vi "rsscope_core_global.vi"() -> ()   [LabVIEW 2014] (continued)
"Read Callback"="", "Write Callback"="", "Supported Models"="", "Instrument Options"="", "Flags"=0, "Help"="Selects the operation type to be performed on the selected operands for the spectrum arithmetic measurement.\n\nAvailable Repeated Capabilities:\nMeasurement: Meas1, Meas2, Meas3, Meas4, Meas5, Meas6, Meas7, Meas8, Meas9, Meas10\r\n\nRemote-control command(s):\nMEASurement<m>:SPECtrum:ARIThmetic:OPERator"}, {"Level"=4, "Class Only"=FALSE, "Identifier"="RSSCOPE_ATTR_SPECTRUM_ARITHMETIC_CONSTANT", "Descriptive Name"="Spectrum Arithmetic Constant", "Data Type"=1, "Command"="MEAS{Measurement}:SPEC:ARIT:CONS", "Access"=2, "Range Table"="RsScope_rngArithmeticConstant", "Read Callback"="", "Write Callback"="", "Supported Models"="", "Instrument Options"="", "Flags"=0, "Help"="Sets a constant numeric value as the second operand of the spectrum arithmetic measurement.\n\nAvailable Repeated Capabilities:\nMeasurement: Meas1, Meas2, Meas3, Meas4, Meas5, Meas6, Meas7, Meas8, Meas9, Meas10\r\n\nRemote-control command(s):\nMEASurement<m>:SPECtrum:ARIThmetic:CONStant"}, {"Level"=4, "Class Only"=FALSE, "Identifier"="RSSCOPE_ATTR_SPECTRUM_ARITHMETIC_CONSTANT_UNIT", "Descriptive Name"="Spectrum Arithmetic Constant Unit", "Data Type"=0, "Command"="MEAS{Measurement}:SPEC:ARIT:COUN", "Access"=2, "Range Table"="RsScope_rngArithmeticOperationType", "Read Callback"="", "Write Callback"="", "Supported Models"="", "Instrument Options"="", "Flags"=0, "Help"="Selects the operation type to be performed on the selected operands for the amplitude/time arithmetic measurement.\n\nAvailable Repeated Capabilities:\nMeasurement: Meas1, Meas2, Meas3, Meas4, Meas5, Meas6, Meas7, Meas8, Meas9, Meas10\r\n\nRemote-control command(s):\nMEASurement<m>:SPECtrum:ARIThmetic:COUNit"}, {"Level"=4, "Class Only"=FALSE, "Identifier"="RSSCOPE_ATTR_SPECTRUM_ARITHMETIC_CUSTOM_NAME_ENABLED", "Descriptive Name"="Spectrum Arithmetic Custom Name Enabled", "Data Type"=3, "Command"="MEAS{Measurement}:SPEC:ARIT:CUNS", "Access"=2, "Range Table"="", "Read Callback"="", "Write Callback"="", "Supported Models"="", "Instrument Options"="", "Flags"=0, "Help"="Enables the use of user-defined custom name for the spectrum arithmetic measurement.\n\nAvailable Repeated Capabilities:\nMeasurement: Meas1, Meas2, Meas3, Meas4, Meas5, Meas6, Meas7, Meas8, Meas9, Meas10\r\n\nRemote-control command(s):\nMEASurement<m>:SPECtrum:ARIThmetic:CUNState"}, {"Level"=4, "Class Only"=FALSE, "Identifier"="RSSCOPE_ATTR_SPECTRUM_ARITHMETIC_CUSTOM_UNIT_ENABLED", "Descriptive Name"="Spectrum Arithmetic Custom Unit Enabled", "Data Type"=3, "Command"="MEAS{Measurement}:SPEC:ARIT:CUUS", "Access"=2, "Range Table"="", "Read Callback"="", "Write Callback"="", "Supported Models"="", "Instrument Options"="", "Flags"=0, "Help"="Enables the use of user-defined custom unit for the amplitude/time arithmetic measurement. You can set the unit with RSSCOPE_ATTR_SPECTRUM_ARITHMETIC_CUSTOM_UNIT.\n\nAvailable Repeated Capabilities:\nMeasurement: Meas1, Meas2, Meas3, Meas4, Meas5, Meas6, Meas7, Meas8, Meas9, Meas10\r\n\nRemote-control command(s):\nMEASurement<m>:SPECtrum:ARIThmetic:CUUState"}, {"Level"=4, "Class Only"=FALSE, "Identifier"="RSSCOPE_ATTR_SPECTRUM_ARITHMETIC_CUSTOM_UNIT", "Descriptive Name"="Spectrum Arithmetic Custom Unit", "Data Type"=2, "Command"="MEAS{Measurement}:SPEC:ARIT:CUUN", "Access"=2, "Range Table"="", "Read Callback"="", "Write Callback"="", "Supported Models"="", "Instrument Options"="", "Flags"=0, "Help"="Sets a user-defined value of the unit for the spectrum arithmetic measurement.\n\nAvailable Repeated Capabilities:\nMeasurement: Meas1, Meas2, Meas3, Meas4, Meas5, Meas6, Meas7, Meas8, Meas9, Meas10\r\n\nRemote-control command(s):\nMEASurement<m>:SPECtrum:ARIThmetic:CUUNit"}, {"Level"=2, "Class Only"=TRUE, "Identifier"="", "Descriptive Name"="Statistics And Long-term Measurement", "Data Type"=0, "Command"="", "Access"=0, "Range Table"="", "Read Callback"="", "Write Callback"="", "Supported Models"="", "Instrument Options"="", "Flags"=0, "Help"="Statistics And Long-term Measurement configures long term measurements, including statistics and measurement histogram over a longer period of time."}, {"Level"=3, "Class Only"=FALSE, "Identifier"="RSSCOPE_ATTR_STATISTICS_ENABLED", "Descriptive Name"="Statistics Enabled", "Data Type"=3, "Command"="MEAS{Measurement}:STAT", "Access"=2, "Range Table"="", "Read Callback"="", "Write Callback"="", "Supported Models"="", "Instrument Options"="", "Flags"=0, "Help"="Enables statistics calculation for the measurement. For RTE the statistics can only be switched globally for all measurements.\n\nAvailable Repeated Capabilities:\nMeasurement: Meas1, Meas2, Meas3, Meas4, Meas5, Meas6, Meas7, Meas8, Meas9, Meas10\r\n\nRemote-control command(s):\nMEASurement<m>:STATistics[:ENABle]"}, {"Level"=3, "Class Only"=FALSE, "Identifier"="RSSCOPE_ATTR_STATISTICS_HISTOGRAM_ENABLED", "Descriptive Name"="Statistics Histogram Enabled", "Data Type"=3, "Command"="MEAS{Measurement}:STAT:HIST", "Access"=2, "Range Table"="", "Read Callback"="", "Write Callback"="", "Supported Models"="", "Instrument Options"="", "Flags"=0, "Help"="Displays histogram of the statistical results. Enabling the histogram enables also the calculation and display of statistics for the measurement results if statistics were disabled. The histogram shows the cumulative occurence distribution of mean measurement results in a graphic.\n\nAvailable Repeated Capabilities:\nMeasurement: Meas1, Meas2, Meas3, Meas4, Meas5, Meas6, Meas7, Meas8, Meas9, Meas10\r\n\nRemote-control command(s):\nMEASurement<m>:STATistics:HISTogram"}, {"Level"=3, "Class Only"=FALSE, "Identifier"="RSSCOPE_ATTR_STATISTICS_RESET_MODE", "Descriptive Name"="Statistics Reset Mode", "Data Type"=0, "Command"="MEAS{Measurement}:STAT:MODE", "Access"=2, "Range Table"="rsscope_rngStatisticsMode", "Read Callback"="", "Write Callback"="", "Supported Models"="", "Instrument Options"="", "Flags"=0, "Help"="Defines when the statistics for long term measurements are reset.\n\nAvailable Repeated Capabilities:\nMeasurement: Meas1, Meas2, Meas3, Meas4, Meas5, Meas6, Meas7, Meas8, Meas9, Meas10\r\n\nRemote-control command(s):\nMEASurement<m>:STATistics:MODE"}, {"Level"=3, "Class Only"=FALSE, "Identifier"="RSSCOPE_ATTR_STATISTICS_RESET_COUNT", "Descriptive Name"="Statistics Reset Count", "Data Type"=0, "Command"="MEAS{Measurement}:STAT:RCO", "Access"=2, "Range Table"="rsscope_rngResetCount", "Read Callback"="", "Write Callback"="", "Supported Models"="", "Instrument Options"="", "Flags"=0, "Help"="Defines the number of measurements after which the statistics are reset.\n\nAvailable Repeated Capabilities:\nMeasurement: Meas1, Meas2, Meas3, Meas4, Meas5, Meas6, Meas7, Meas8, Meas9, Meas10\r\n\nRemote-control command(s):\nMEASurement<m>:STATistics:RCOunt"}, {"Level"=3, "Class Only"=FALSE, "Identifier"="RSSCOPE_ATTR_STATISTICS_RESET_TIME", "Descriptive Name"="Statistics Reset Time", "Data Type"=1, "Command"="MEAS{Measurement}:STAT:RTIM", "Access"=2, "Range Table"="rsscope_rngResetTime", "Read Callback"="", "Write Callback"="", "Supported Models"="", "Instrument Options"="", "Flags"=0, "Help"="Defines the time or period after which the statistics are reset.\n\nAvailable Repeated Capabilities:\nMeasurement: Meas1, Meas2, Meas3, Meas4, Meas5, Meas6, Meas7, Meas8, Meas9, Meas10\r\n\nRemote-control command(s):\nMEASurement<m>:STATistics:RTIMe"}, {"Level"=3, "Class Only"=FALSE, "Identifier"="RSSCOPE_ATTR_STATISTICS_RESET_MEASUREMENTS_COUNT", "Descriptive Name"="Statistics Reset Measurements Count", "Data Type"=0, "Command"="MEAS{Measurement}:STAT:RME", "Access"=2, "Range Table"="rsscope_rngStatisticsMeasurementsCount", "Read Callback"="", "Write Callback"="", "Supported Models"="", "Instrument Options"="", "Flags"=0, "Help"="Defines the number of measurement results from which one point of the long term measurement is created.\n\nAvailable Repeated Capabilities:\nMeasurement: Meas1, Meas2, Meas3, Meas4, Meas5, Meas6, Meas7, Meas8, Meas9, Meas10\r\n\nRemote-control command(s):\nMEASurement<m>:STATistics:RMEascount"}, {"Level"=3, "Class Only"=FALSE, "Identifier"="RSSCOPE_ATTR_STATISTICS_RESET", "Descriptive Name"="Statistics Reset", "Data Type"=4, "Command"="MEAS{Measurement}:STAT:RES", "Access"=1, "Range Table"="", "Read Callback"="", "Write Callback"="", "Supported Models"="", "Instrument Options"="", "Flags"=0, "Help"="Resets the statistics.\n\nAvailable Repeated Capabilities:\nMeasurement: Meas1, Meas2, Meas3, Meas4, Meas5, Meas6, Meas7, Meas8, Meas9, Meas10\r\n\nRemote-control command(s):\nMEASurement<m>:STATistics:RESet"}, {"Level"=3, "Class Only"=FALSE, "Identifier"="RSSCOPE_ATTR_STATISTICS_NUMBER_OF_BINS", "Descriptive Name"="Statistics Number Of Bins", "Data Type"=0, "Command"="MEAS{Measurement}:STAT:HBIN", "Access"=2, "Range Table"="RsScope_rngStatisticsNumberOfBins", "Read Callback"="", "Write Callback"="", "Supported Models"="", "Instrument Options"="", "Flags"=0, "Help"="Sets the number of bins - the number of vertical bars that build the histogram. If &apos;Continuous auto scale&apos; is enabled, the instrument determines the number of bins based on the time base, the current measurements, and other settings. To set the number of bins manually, disable &apos;Continuous auto scale&apos;.\n\nAvailable Repeated Capabilities:\nMeasurement: Meas1, Meas2, Meas3, Meas4, Meas5, Meas6, Meas7, Meas8, Meas9, Meas10\r\n\nRemote-control command(s):\nMEASurement<m>:STATistics:HBINs"}, {"Level"=3, "Class Only"=FALSE, "Identifier"="RSSCOPE_ATTR_TRACK_ENABLED", "Descriptive Name"="Track Enabled", "Data Type"=3, "Command"="MEAS{Measurement}:TRAC", "Access"=2, "Range Table"="", "Read Callback"="", "Write Callback"="", "Supported Models"="", "Instrument Options"="", "Flags"=0, "Help"="Enables or disables the track of the indicated channel.\n\nAvailable Repeated Capabilities:\nMeasurement: Meas1, Meas2, Meas3, Meas4, Meas5, Meas6, Meas7, Meas8, Meas9, Meas10\r\n\nRemote-control command(s):\nMEASurement<m>:TRACk[:STATe]"}, {"Level"=3, "Class Only"=FALSE, "Identifier"="RSSCOPE_ATTR_PROTOCOL_AUDIO_TRACK_ENABLED", "Descriptive Name"="Protocol Audio Track Enabled", "Data Type"=3, "Command"="MEAS{Measurement}:TRAC", "Access"=2, "Range Table"="", "Read Callback"="", "Write Callback"="", "Supported Models"="", "Instrument Options"="", "Flags"=0, "Help"="Enables or disables the track of the indicated channel.\n\nAvailable Repeated Capabilities:\nMeasurement: Meas1, Meas2, Meas3, Meas4, Meas5, Meas6, Meas7, Meas8, Meas9, Meas10\r\n\nRemote-control command(s):\nMEASurement<m>:TRACk[:STATe]"}, {"Level"=3, "Class Only"=FALSE, "Identifier"="RSSCOPE_ATTR_TRACK_WAVEFORM_HEADER", "Descriptive Name"="Track Waveform Header", "Data Type"=2, "Command"="MEAS{Measurement}:TRAC:DATA:HEAD?", "Access"=0, "Range Table"="", "Read Callback"="", "Write Callback"="", "Supported Models"="", "Instrument Options"="", "Flags"=0, "Help"="Returns the header of the track.\n\nAvailable Repeated Capabilities:\nMeasurement: Meas1, Meas2, Meas3, Meas4, Meas5, Meas6, Meas7, Meas8, Meas9, Meas10\r\n\nRemote-control command(s):\nMEASurement<m>:TRACk:DATA:HEADer?"}, {"Level"=3, "Class Only"=FALSE, "Identifier"="RSSCOPE_ATTR_TRACK_WAVEFORM_DATA_TYPE", "Descriptive Name"="Track Waveform Data Type", "Data Type"=2, "Command"="MEAS{Measurement}:TRAC:DATA:STYP?", "Access"=0, "Range Table"="", "Read Callback"="", "Write Callback"="", "Supported Models"="", "Instrument Options"="", "Flags"=0, "Help"="Returns the data type.\n\nAvailable Repeated Capabilities:\nMeasurement: Meas1, Meas2, Meas3, Meas4, Meas5, Meas6, Meas7, Meas8, Meas9, Meas10\r\n\nRemote-control command(s):\nMEASurement<m>:TRACk:DATA:STYPe?"}, {"Level"=3, "Class Only"=FALSE, "Identifier"="RSSCOPE_ATTR_PROTOCOL_AUDIO_TRACK_WAVEFORM_DATA_TYPE", "Descriptive Name"="Protocol Audio Track Waveform Data Type", "Data Type"=2, "Command"="MEAS{Measurement}:TRAC:DATA:STYP?", "Access"=0, "Range Table"="", "Read Callback"="", "Write Callback"="", "Supported Models"="", "Instrument Options"="", "Flags"=0, "Help"="Returns the data type.\n\nAvailable Repeated Capabilities:\nMeasurement: Meas1, Meas2, Meas3, Meas4, Meas5, Meas6, Meas7, Meas8, Meas9, Meas10\r\n\nRemote-control command(s):\nMEASurement<m>:TRACk:DATA:STYPe?"}, {"Level"=3, "Class Only"=FALSE, "Identifier"="RSSCOPE_ATTR_LONG_TERM_MEASUREMENT_ENABLED", "Descriptive Name"="Long Term Measurement Enabled", "Data Type"=3, "Command"="MEAS{Measurement}:LTM", "Access"=2, "Range Table"="", "Read Callback"="", "Write Callback"="", "Supported Models"="", "Instrument Options"="", "Flags"=0, "Help"="Enables long term measurement for a defined number of measurement points or a specified time.\n\nAvailable Repeated Capabilities:\nMeasurement: Meas1, Meas2, Meas3, Meas4, Meas5, Meas6, Meas7, Meas8, Meas9, Meas10\r\n\nRemote-control command(s):\nMEASurement<m>:LTMeas[:STATe]"}, {"Level"=3, "Class Only"=FALSE, "Identifier"="RSSCOPE_ATTR_LONG_TERM_COUNT", "Descriptive Name"="Long Term Count", "Data Type"=0, "Command"="MEAS{Measurement}:LTM:COUN", "Access"=2, "Range Table"="rsscope_rngLongTermCount", "Read Callback"="", "Write Callback"="", "Supported Models"="", "Instrument Options"="", "Flags"=0, "Help"="Defines the total number of points to be measured during the long term measurement.\n\nAvailable Repeated Capabilities:\nMeasurement: Meas1, Meas2, Meas3, Meas4, Meas5, Meas6, Meas7, Meas8, Meas9, Meas10\r\n\nRemote-control command(s):\nMEASurement<m>:LTMeas:COUNt"}, {"Level"=3, "Class Only"=FALSE, "Identifier"="RSSCOPE_ATTR_LONG_TERM_DURATION", "Descriptive Name"="Long Term Duration", "Data Type"=0, "Command"="MEAS{Measurement}:LTM:TIME", "Access"=2, "Range Table"="", "Read Callback"="", "Write Callback"="", "Supported Models"="", "Instrument Options"="", "Flags"=0, "Help"="Defines the total duration of the long term measurement.\n\nAvailable Repeated Capabilities:\nMeasurement: Meas1, Meas2, Meas3, Meas4, Meas5, Meas6, Meas7, Meas8, Meas9, Meas10\r\n\nRemote-control command(s):\nMEASurement<m>:LTMeas:TIME"}, {"Level"=3, "Class Only"=FALSE, "Identifier"="RSSCOPE_ATTR_LONG_TERM_VERTICAL_OFFSET", "Descriptive Name"="Long Term Vertical Offset", "Data Type"=1, "Command"="MEAS{Measurement}:VERT:OFFS", "Access"=2, "Range Table"="", "Read Callback"="", "Write Callback"="", "Supported Models"="", "Instrument Options"="", "Flags"=0, "Help"="Defines a vertical offset for the long term measurement.\n\nAvailable Repeated Capabilities:\nMeasurement: Meas1, Meas2, Meas3, Meas4, Meas5, Meas6, Meas7, Meas8, Meas9, Meas10\r\n\nRemote-control command(s):\nMEASurement<m>:VERTical:OFFSet"}, {"Level"=3, "Class Only"=FALSE, "Identifier"="RSSCOPE_ATTR_LONG_TERM_VERTICAL_SCALING", "Descriptive Name"="Long Term Vertical Scaling", "Data Type"=1, "Command"="MEAS{Measurement}:VERT:SCAL", "Access"=2, "Range Table"="RsScope_rngLongTermVerticalScaling", "Read Callback"="", "Write Callback"="", "Supported Models"="", "Instrument Options"="", "Flags"=0, "Help"="Defines the vertical scaling per division, so that the scaling can be adapted automatically during the long term measurement period.\n\nAvailable Repeated Capabilities:\nMeasurement: Meas1, Meas2, Meas3, Meas4, Meas5, Meas6, Meas7, Meas8, Meas9, Meas10\r\n\nRemote-control command(s):\nMEASurement<m>:VERTical:SCALe"}, {"Level"=3, "Class Only"=FALSE, "Identifier"="RSSCOPE_ATTR_LONG_TERM_VERTICAL_CONTINUOUS_AUTO_SCALING", "Descriptive Name"="Long Term Vertical Continuous Auto Scaling", "Data Type"=3, "Command"="MEAS{Measurement}:VERT:CONT", "Access"=2, "Range Table"="", "Read Callback"="", "Write Callback"="", "Supported Models"="", "Instrument Options"="", "Flags"=0, "Help"="If enabled, automatic vertical scaling is performed whenever the waveform does not fit in the diagram during the long term measurement period.\n\nAvailable Repeated Capabilities:\nMeasurement: Meas1, Meas2, Meas3, Meas4, Meas5, Meas6, Meas7, Meas8, Meas9, Meas10\r\n\nRemote-control command(s):\nMEASurement<m>:VERTical:CONT"}, {"Level"=3, "Class Only"=FALSE, "Identifier"="RSSCOPE_ATTR_LONG_TERM_VERTICAL_AUTOSCALE", "Descriptive Name"="Long Term Vertical Autoscale", "Data Type"=4, "Command"="MEAS{Measurement}:VERT:AUTO", "Access"=1, "Range Table"="", "Read Callback"="", "Write Callback"="", "Supported Models"="", "Instrument Options"="", "Flags"=0, "Help"="If enabled, vertical scaling is adapted to the current measurement results automatically during the long term measurement period.\n\nAvailable Repeated Capabilities:\nMeasurement: Meas1, Meas2, Meas3, Meas4, Meas5, Meas6, Meas7, Meas8, Meas9, Meas10\r\n\nRemote-control command(s):\nMEASurement<m>:VERTical:AUTO"}, {"Level"=3, "Class Only"=FALSE, "Identifier"="RSSCOPE_ATTR_LONG_TERM_ENVIRONMENT_SENSOR_ENABLED", "Descriptive Name"="Long Term Environment Sensor Enabled", "Data Type"=3, "Command"="MEAS{Measurement}:LTM:ENVS:STAT", "Access"=2, "Range Table"="", "Read Callback"="", "Write Callback"="", "Supported Models"="", "Instrument Options"="", "Flags"=0, "Help"="Enables the evaluation of a connected environment sensor.\n\nAvailable Repeated Capabilities:\nMeasurement: Meas1, Meas2, Meas3, Meas4, Meas5, Meas6, Meas7, Meas8, Meas9, Meas10\r\n\nRemote-control command(s):\nMEASurement<m>:LTMeas:ENVSensor:STATe"}, {"Level"=2, "Class Only"=TRUE, "Identifier"="", "Descriptive Name"="Protocol", "Data Type"=0, "Command"="", "Access"=0, "Range Table"="", "Read Callback"="", "Write Callback"="", "Supported Models"="", "Instrument Options"="", "Flags"=0, "Help"="This class contains methods for configuring and measuring protocol measurements. Before starting the protocol measurement a bus type has to be selected (RSSCOPE_ATTR_PROTOCOL_TYPE) and the bus has to be activated (RSSCOPE_ATTR_PROTOCOL_STATE)."}, {"Level"=3, "Class Only"=FALSE, "Identifier"="RSSCOPE_ATTR_PROTOCOL_MAIN_MEASUREMENT", "Descriptive Name"="Protocol Main Measurement", "Data Type"=0, "Command"="MEAS{Measurement}:MAIN", "Access"=2, "Range Table"="rsscope_rngProtocolMeasurementType", "Read Callback"="", "Write Callback"="", "Supported Models"="", "Instrument Options"="K35", "Flags"=0, "Help"="Defines or queries the main measurement. This measurement is the one referred to if the measurement waveform is used as a source for math calculations. The main measurement type must belong to the same category as the other types assigned to the same measurement waveform, if there are any.\n\nAvailable Repeated Capabilities:\nMeasurement: Meas1, Meas2, Meas3, Meas4, Meas5, Meas6, Meas7, Meas8, Meas9, Meas10\r\n\nRemote-control command(s):\nMEASurement<m>:MAIN"}, {"Level"=3, "Class Only"=FALSE, "Identifier"="RSSCOPE_ATTR_PROTOCOL_ADDITIONAL_MEASUREMENT", "Descriptive Name"="Protocol Additional Measurement", "Data Type"=6, "Command"="MEAS{Measurement}:ADD", "Access"=1, "Range Table"="", "Read Callback"="", "Write Callback"="", "Supported Models"="", "Instrument Options"="K35", "Flags"=0, "Help"="Adds additional measurements to the indicated measurement group. Only one measurement can be enabled or disabled per command. The query returns the state of the specified measurement.\n\nNote that each measurement group must contain measurements from the same category. For example, if the main measurement of measurement group 1 is amplitude, then you cannot enable an eye width measurementin the same measurement group.\n\nAvailable Repeated Capabilities:\nMeasurement: Meas1, Meas2, Meas3, Meas4, Meas5, Meas6, Meas7, Meas8, Meas9, Meas10\r\n\nRemote-control command(s):\nMEASurement<m>:ADDitional"}, {"Level"=3, "Class Only"=FALSE, "Identifier"="RSSCOPE_ATTR_FRAME_TO_FRAME_FROM_FRAME", "Descriptive Name"="Frame To Frame From Frame", "Data Type"=2, "Command"="MEAS{Measurement}:PROT:F2FR:FRMF", "Access"=2, "Range Table"="", "Read Callback"="", "Write Callback"="", "Supported Models"="", "Instrument Options"="", "Flags"=0, "Help"="Sets the type of start frame for the frame to frame protocol measurement. Valid values vary by protocol.\n\nAvailable Repeated Capabilities:\nMeasurement: Meas1, Meas2, Meas3, Meas4, Meas5, Meas6, Meas7, Meas8, Meas9, Meas10\r\n\nRemote-control command(s):\nMEASurement<m>:PROTocol:F2FRame:FRMFrom"}, {"Level"=3, "Class Only"=FALSE, "Identifier"="RSSCOPE_ATTR_FRAME_TO_FRAME_FROM_FIELD", "Descriptive Name"="Frame To Frame From Field", "Data Type"=2, "Command"="MEAS{Measurement}:PROT:F2FR:FLDF", "Access"=2, "Range Table"="", "Read Callback"="", "Write Callback"="", "Supported Models"="", "Instrument Options"="", "Flags"=0, "Help"="Sets the type of field for the start frame of the frame to frame protocol measurement. Valid values vary by frame.\n\nAvailable Repeated Capabilities:\nMeasurement: Meas1, Meas2, Meas3, Meas4, Meas5, Meas6, Meas7, Meas8, Meas9, Meas10\r\n\nRemote-control command(s):\nMEASurement<m>:PROTocol:F2FRame:FLDFrom"}, {"Level"=3, "Class Only"=FALSE, "Identifier"="RSSCOPE_ATTR_FRAME_TO_FRAME_FROM_VALUE", "Descriptive Name"="Frame To Frame From Value", "Data Type"=2, "Command"="MEAS{Measurement}:PROT:F2FR:VALF", "Access"=2, "Range Table"="", "Read Callback"="", "Write Callback"="", "Supported Models"="", "Instrument Options"="", "Flags"=0, "Help"="Sets the field value of the start frame for the frame to frame protocol measurement.\n\nAvailable Repeated Capabilities:\nMeasurement: Meas1, Meas2, Meas3, Meas4, Meas5, Meas6, Meas7, Meas8, Meas9, Meas10\r\n\nRemote-control command(s):\nMEASurement<m>:PROTocol:F2FRame:VALFrom"}, {"Level"=3, "Class Only"=FALSE, "Identifier"="RSSCOPE_ATTR_FRAME_TO_FRAME_TO_FRAME", "Descriptive Name"="Frame To Frame To Frame", "Data Type"=2, "Command"="MEAS{Measurement}:PROT:F2FR:FRMT", "Access"=2, "Range Table"="", "Read Callback"="", "Write Callback"="", "Supported Models"="", "Instrument Options"="", "Flags"=0, "Help"="Sets the type of end frame for the frame to frame protocol measurement. Valid values vary by protocol.\n\nAvailable Repeated Capabilities:\nMeasurement: Meas1, Meas2, Meas3, Meas4, Meas5, Meas6, Meas7, Meas8, Meas9, Meas10\r\n\nRemote-control command(s):\nMEASurement<m>:PROTocol:F2FRame:FRMTo"}, {"Level"=3, "Class Only"=FALSE, "Identifier"="RSSCOPE_ATTR_FRAME_TO_FRAME_TO_FIELD", "Descriptive Name"="Frame To Frame To Field", "Data Type"=2, "Command"="MEAS{Measurement}:PROT:F2FR:FLDT", "Access"=2, "Range Table"="", "Read Callback"="", "Write Callback"="", "Supported Models"="", "Instrument Options"="", "Flags"=0, "Help"="Sets the type of field for the end frame of the frame to frame protocol measurement. Valid values vary by frame.\n\nAvailable Repeated Capabilities:\nMeasurement: Meas1, Meas2, Meas3, Meas4, Meas5, Meas6, Meas7, Meas8, Meas9, Meas10\r\n\nRemote-control command(s):\nMEASurement<m>:PROTocol:F2FRame:FLDTo"}, {"Level"=3, "Class Only"=FALSE, "Identifier"="RSSCOPE_ATTR_FRAME_TO_FRAME_TO_VALUE", "Descriptive Name"="Frame To Frame To Value", "Data Type"=2, "Command"="MEAS{Measurement}:PROT:F2FR:VALT", "Access"=2, "Range Table"="", "Read Callback"="", "Write Callback"="", "Supported Models"="", "Instrument Options"="", "Flags"=0, "Help"="Sets the field value of the end frame for the frame to frame protocol measurement.\n\nAvailable Repeated Capabilities:\nMeasurement: Meas1, Meas2, Meas3, Meas4, Meas5, Meas6, Meas7, Meas8, Meas9, Meas10\r\n\nRemote-control command(s):\nMEASurement<m>:PROTocol:F2FRame:VALTo"}, {"Level"=3, "Class Only"=FALSE, "Identifier"="RSSCOPE_ATTR_TRIGGER_TO_FRAME_DIRECTION", "Descriptive Name"="Trigger To Frame Direction", "Data Type"=0, "Command"="MEAS{Measurement}:PROT:T2FR:DIR", "Access"=2, "Range Table"="RsScope_rngTriggerToFrameDirection", "Read Callback"="", "Write Callback"="", "Supported Models"="", "Instrument Options"="", "Flags"=0, "Help"="Sets the direction of the field for trigger to frame protocol measurement.\n\nAvailable Repeated Capabilities:\nMeasurement: Meas1, Meas2, Meas3, Meas4, Meas5, Meas6, Meas7, Meas8, Meas9, Meas10\r\n\nRemote-control command(s):\nMEASurement<m>:PROTocol:T2FRame:DIRection"}, {"Level"=3, "Class Only"=FALSE, "Identifier"="RSSCOPE_ATTR_TRIGGER_TO_FRAME_FRAME", "Descriptive Name"="Trigger To Frame Frame", "Data Type"=2, "Command"="MEAS{Measurement}:PROT:T2FR:FRM", "Access"=2, "Range Table"="", "Read Callback"="", "Write Callback"="", "Supported Models"="", "Instrument Options"="", "Flags"=0, "Help"="Sets the value of the frame for trigger to frame protocol measurement. Valid values vary by protocol.\n\nAvailable Repeated Capabilities:\nMeasurement: Meas1, Meas2, Meas3, Meas4, Meas5, Meas6, Meas7, Meas8, Meas9, Meas10\r\n\nRemote-control command(s):\nMEASurement<m>:PROTocol:T2FRame:FRM"}, {"Level"=3, "Class Only"=FALSE, "Identifier"="RSSCOPE_ATTR_TRIGGER_TO_FRAME_FIELD", "Descriptive Name"="Trigger To Frame Field", "Data Type"=2, "Command"="MEAS{Measurement}:PROT:T2FR:FLD", "Access"=2, "Range Table"="", "Read Callback"="", "Write Callback"="", "Supported Models"="", "Instrument Options"="", "Flags"=0, "Help"="Sets the type of the field for trigger to frame protocol measurement. Valid values vary by frame.\n\nAvailable Repeated Capabilities:\nMeasurement: Meas1, Meas2, Meas3, Meas4, Meas5, Meas6, Meas7, Meas8, Meas9, Meas10\r\n\nRemote-control command(s):\nMEASurement<m>:PROTocol:T2FRame:FLD"}, {"Level"=3, "Class Only"=FALSE, "Identifier"="RSSCOPE_ATTR_TRIGGER_TO_FRAME_VALUE", "Descriptive Name"="Trigger To Frame Value", "Data Type"=2, "Command"="MEAS{Measurement}:PROT:T2FR:VAL", "Access"=2, "Range Table"="", "Read Callback"="", "Write Callback"="", "Supported Models"="", "Instrument Options"="", "Flags"=0, "Help"="Sets the value of the field for trigger to frame protocol measurement.\n\nAvailable Repeated Capabilities:\nMeasurement: Meas1, Meas2, Meas3, Meas4, Meas5, Meas6, Meas7, Meas8, Meas9, Meas10\r\n\nRemote-control command(s):\nMEASurement<m>:PROTocol:T2FRame:VALue"}, {"Level"=3, "Class Only"=FALSE, "Identifier"="RSSCOPE_ATTR_FIELD_VALUE_FRAME_IDENTIFICATION_FRAME", "Descriptive Name"="Field Value Frame Identification Frame", "Data Type"=2, "Command"="MEAS{Measurement}:PROT:FLDV:FRM", "Access"=2, "Range Table"="", "Read Callback"="", "Write Callback"="", "Supported Models"="", "Instrument Options"="", "Flags"=0, "Help"="Sets the type frame for the field value protocol measurement. Valid values vary by protocol.\n\nAvailable Repeated Capabilities:\nMeasurement: Meas1, Meas2, Meas3, Meas4, Meas5, Meas6, Meas7, Meas8, Meas9, Meas10\r\n\nRemote-control command(s):\nMEASurement<m>:PROTocol:FLDValue:FRM"}, {"Level"=3, "Class Only"=FALSE, "Identifier"="RSSCOPE_ATTR_FIELD_VALUE_FRAME_IDENTIFICATION_FIELD", "Descriptive Name"="Field Value Frame Identification Field", "Data Type"=2, "Command"="MEAS{Measurement}:PROT:FLDV:FLD", "Access"=2, "Range Table"="", "Read Callback"="", "Write Callback"="", "Supported Models"="", "Instrument Options"="", "Flags"=0, "Help"="Sets the type of field for the frame of the field value protocol measurement. Valid values vary by frame.\n\nAvailable Repeated Capabilities:\nMeasurement: Meas1, Meas2, Meas3, Meas4, Meas5, Meas6, Meas7, Meas8, Meas9, Meas10\r\n\nRemote-control command(s):\nMEASurement<m>:PROTocol:FLDValue:FLD"}, {"Level"=3, "Class Only"=FALSE, "Identifier"="RSSCOPE_ATTR_FIELD_VALUE_FRAME_IDENTIFICATION_VALUE", "Descriptive Name"="Field Value Frame Identification Value", "Data Type"=2, "Command"="MEAS{Measurement}:PROT:FLDV:VAL", "Access"=2, "Range Table"="", "Read Callback"="", "Write Callback"="", "Supported Models"="", "Instrument Options"="", "Flags"=0, "Help"="Sets the field value of the frame for the field value protocol measurement.\n\nAvailable Repeated Capabilities:\nMeasurement: Meas1, Meas2, Meas3, Meas4, Meas5, Meas6, Meas7, Meas8, Meas9, Meas10\r\n\nRemote-control command(s):\nMEASurement<m>:PROTocol:FLDValue:VALue"}, {"Level"=3, "Class Only"=FALSE, "Identifier"="RSSCOPE_ATTR_FIELD_VALUE_FIELD_TO_BE_TRACKED", "Descriptive Name"="Field Value Field To Be Tracked", "Data Type"=2, "Command"="MEAS{Measurement}:PROT:FLDV:TRCK", "Access"=2, "Range Table"="", "Read Callback"="", "Write Callback"="", "Supported Models"="", "Instrument Options"="", "Flags"=0, "Help"="Sets the field to be tracked value of the frame for the field value protocol measurement.\n\nAvailable Repeated Capabilities:\nMeasurement: Meas1, Meas2, Meas3, Meas4, Meas5, Meas6, Meas7, Meas8, Meas9, Meas10\r\n\nRemote-control command(s):\nMEASurement<m>:PROTocol:FLDValue:TRCK"}, {"Level"=3, "Class Only"=FALSE, "Identifier"="RSSCOPE_ATTR_MAIN_BIT_RATE_FRAME_NAME", "Descriptive Name"="Main Bit Rate Frame Name", "Data Type"=2, "Command"="MEAS{Measurement}:PROT:MBIT:FRM", "Access"=2, "Range Table"="", "Read Callback"="", "Write Callback"="", "Supported Models"="", "Instrument Options"="", "Flags"=0, "Help"="Sets the type frame for the main bit rate protocol measurement.\n\nAvailable Repeated Capabilities:\nMeasurement: Meas1, Meas2, Meas3, Meas4, Meas5, Meas6, Meas7, Meas8, Meas9, Meas10\r\n\nRemote-control command(s):\nMEASurement<m>:PROTocol:MBITrate:FRM"}, {"Level"=3, "Class Only"=FALSE, "Identifier"="RSSCOPE_ATTR_MAIN_BIT_RATE_FIELD_NAME", "Descriptive Name"="Main Bit Rate Field Name", "Data Type"=2, "Command"="MEAS{Measurement}:PROT:MBIT:FLD", "Access"=2, "Range Table"="", "Read Callback"="", "Write Callback"="", "Supported Models"="", "Instrument Options"="", "Flags"=0, "Help"="Sets the type of field for the frame of the main bit rate protocol measurement.\n\nAvailable Repeated Capabilities:\nMeasurement: Meas1, Meas2, Meas3, Meas4, Meas5, Meas6, Meas7, Meas8, Meas9, Meas10\r\n\nRemote-control command(s):\nMEASurement<m>:PROTocol:MBITrate:FLD"}, {"Level"=3, "Class Only"=FALSE, "Identifier"="RSSCOPE_ATTR_MAIN_BIT_RATE_ID_VALUE", "Descriptive Name"="Main Bit Rate ID Value", "Data Type"=6, "Command"="MEAS{Measurement}:PROT:MBIT:VAL", "Access"=2, "Range Table"="", "Read Callback"="", "Write Callback"="", "Supported Models"="", "Instrument Options"="", "Flags"=0, "Help"="Sets the field value of the frame for the main bit rate protocol measurement.\n\nNote: Possible to set max up to 8 values of comma separated #HXX,#H01.....\n\nAvailable Repeated Capabilities:\nMeasurement: Meas1, Meas2, Meas3, Meas4, Meas5, Meas6, Meas7, Meas8, Meas9, Meas10\r\n\nRemote-control command(s):\nMEASurement<m>:PROTocol:MBITrate:VAL"}, {"Level"=3, "Class Only"=FALSE, "Identifier"="RSSCOPE_ATTR_SECONDARY_BIT_RATE_FRAME_NAME", "Descriptive Name"="Secondary Bit Rate Frame Name", "Data Type"=2, "Command"="MEAS{Measurement}:PROT:SBIT:FRM", "Access"=2, "Range Table"="", "Read Callback"="", "Write Callback"="", "Supported Models"="", "Instrument Options"="", "Flags"=0, "Help"="Sets the type frame for the secondary bit rate protocol measurement.\n\nAvailable Repeated Capabilities:\nMeasurement: Meas1, Meas2, Meas3, Meas4, Meas5, Meas6, Meas7, Meas8, Meas9, Meas10\r\n\nRemote-control command(s):\nMEASurement<m>:PROTocol:SBITrate:FRM"}, {"Level"=3, "Class Only"=FALSE, "Identifier"="RSSCOPE_ATTR_SECONDARY_BIT_RATE_FIELD_NAME", "Descriptive Name"="Secondary Bit Rate Field Name", "Data Type"=2, "Command"="MEAS{Measurement}:PROT:SBIT:FLD", "Access"=2, "Range Table"="", "Read Callback"="", "Write Callback"="", "Supported Models"="", "Instrument Options"="", "Flags"=0, "Help"="Sets the type of field for the frame of the secondary bit rate protocol measurement.\n\nAvailable Repeated Capabilities:\nMeasurement: Meas1, Meas2, Meas3, Meas4, Meas5, Meas6, Meas7, Meas8, Meas9, Meas10\r\n\nRemote-control command(s):\nMEASurement<m>:PROTocol:SBITrate:FLD"}, {"Level"=3, "Class Only"=FALSE, "Identifier"="RSSCOPE_ATTR_SECONDARY_BIT_RATE_ID_VALUE", "Descriptive Name"="Secondary Bit Rate ID Value", "Data Type"=6, "Command"="MEAS{Measurement}:PROT:SBIT:VAL", "Access"=2, "Range Table"="", "Read Callback"="", "Write Callback"="", "Supported Models"="", "Instrument Options"="", "Flags"=0, "Help"="Sets the field value of the frame for the secondary bit rate protocol measurement.\n\nNote: Possible to set max up to 8 values of comma separated #HXX,#H01....\n\nAvailable Repeated Capabilities:\nMeasurement: Meas1, Meas2, Meas3, Meas4, Meas5, Meas6, Meas7, Meas8, Meas9, Meas10\r\n\nRemote-control command(s):\nMEASurement<m>:PROTocol:SBITrate:VAL"}, {"Level"=2, "Class Only"=TRUE, "Identifier"="", "Descriptive Name"="Gating", "Data Type"=0, "Command"="", "Access"=0, "Range Table"="", "Read Callback"="", "Write Callback"="", "Supported Models"="", "Instrument Options"="", "Flags"=0, "Help"="Defines the measurement gate."}, {"Level"=3, "Class Only"=FALSE, "Identifier"="RSSCOPE_ATTR_GATING_ENABLED", "Descriptive Name"="Gating Enabled", "Data Type"=3, "Command"="MEAS{Measurement}:GATE", "Access"=2, "Range Table"="", "Read Callback"="", "Write Callback"="", "Supported Models"="", "Instrument Options"="", "Flags"=0, "Help"="Considers the gating settings of the source waveform for the measurement.\n\nAvailable Repeated Capabilities:\nMeasurement: Meas1, Meas2, Meas3, Meas4, Meas5, Meas6, Meas7, Meas8, Meas9, Meas10\r\n\nRemote-control command(s):\nMEASurement<m>:GATE[:STATe]"}, {"Level"=3, "Class Only"=FALSE, "Identifier"="RSSCOPE_ATTR_GATING_MODE", "Descriptive Name"="Gating Mode", "Data Type"=0, "Command"="MEAS{Measurement}:GATE:MODE", "Access"=2, "Range Table"="rsscope_rngAbsRel", "Read Callback"="", "Write Callback"="", "Supported Models"="", "Instrument Options"="", "Flags"=0, "Help"="Defines whether the gate settings are configured using absolute or relative values.\n\nAvailable Repeated Capabilities:\nMeasurement: Meas1, Meas2, Meas3, Meas4, Meas5, Meas6, Meas7, Meas8, Meas9, Meas10\r\n\nRemote-control command(s):\nMEASurement<m>:GATE:MODE"}, {"Level"=3, "Class Only"=FALSE, "Identifier"="RSSCOPE_ATTR_GATING_ABSOLUTE_START", "Descriptive Name"="Gating Absolute Start", "Data Type"=1, "Command"="MEAS{Measurement}:GATE:ABS:STAR", "Access"=2, "Range Table"="", "Read Callback"="", "Write Callback"="", "Supported Models"="", "Instrument Options"="", "Flags"=0, "Help"="Define the absolute start values for the gate.\n\nAvailable Repeated Capabilities:\nMeasurement: Meas1, Meas2, Meas3, Meas4, Meas5, Meas6, Meas7, Meas8, Meas9, Meas10\r\n\nRemote-control command(s):\nMEASurement<m>:GATE:ABSolute:STARt"}, {"Level"=3, "Class Only"=FALSE, "Identifier"="RSSCOPE_ATTR_GATING_RELATIVE_START", "Descriptive Name"="Gating Relative Start", "Data Type"=1, "Command"="MEAS{Measurement}:GATE:REL:STAR", "Access"=2, "Range Table"="RsScope_rngPercent", "Read Callback"="", "Write Callback"="", "Supported Models"="", "Instrument Options"="", "Flags"=0, "Help"="Define the relative start values for the gate.\n\nAvailable Repeated Capabilities:\nMeasurement: Meas1, Meas2, Meas3, Meas4, Meas5, Meas6, Meas7, Meas8, Meas9, Meas10\r\n\nRemote-control command(s):\nMEASurement<m>:GATE:RELative:STARt"}, {"Level"=3, "Class Only"=FALSE, "Identifier"="RSSCOPE_ATTR_GATING_ABSOLUTE_STOP", "Descriptive Name"="Gating Absolute Stop", "Data Type"=1, "Command"="MEAS{Measurement}:GATE:ABS:STOP", "Access"=2, "Range Table"="", "Read Callback"="", "Write Callback"="", "Supported Models"="", "Instrument Options"="", "Flags"=0, "Help"="Define the absolute end values for the gate.\n\nAvailable Repeated Capabilities:\nMeasurement: Meas1, Meas2, Meas3, Meas4, Meas5, Meas6, Meas7, Meas8, Meas9, Meas10\r\n\nRemote-control command(s):\nMEASurement<m>:GATE:ABSolute:STOP"}, {"Level"=3, "Class Only"=FALSE, "Identifier"="RSSCOPE_ATTR_GATING_RELATIVE_STOP", "Descriptive Name"="Gating Relative Stop", "Data Type"=1, "Command"="MEAS{Measurement}:GATE:REL:STOP", "Access"=2, "Range Table"="RsScope_rngPercent", "Read Callback"="", "Write Callback"="", "Supported Models"="", "Instrument Options"="", "Flags"=0, "Help"="Define the relative end values for the gate.\n\nAvailable Repeated Capabilities:\nMeasurement: Meas1, Meas2, Meas3, Meas4, Meas5, Meas6, Meas7, Meas8, Meas9, Meas10\r\n\nRemote-control command(s):\nMEASurement<m>:GATE:RELative:STOP"}, {"Level"=3, "Class Only"=FALSE, "Identifier"="RSSCOPE_ATTR_GATING_NOISE", "Descriptive Name"="Gating Noise", "Data Type"=0, "Command"="MEAS{Measurement}:GATE:NOIS", "Access"=2, "Range Table"="rsscope_rngLowUpp", "Read Callback"="", "Write Callback"="", "Supported Models"="", "Instrument Options"="", "Flags"=0, "Help"="Noise evaluation area.\n\nAvailable Repeated Capabilities:\nMeasurement: Meas1, Meas2, Meas3, Meas4, Meas5, Meas6, Meas7, Meas8, Meas9, Meas10\r\n\nRemote-control command(s):\nMEASurement<m>:GATE:NOISe"}, {"Level"=3, "Class Only"=FALSE, "Identifier"="RSSCOPE_ATTR_GATING_SHOW_GATE_AREA", "Descriptive Name"="Gating Show Gate Area", "Data Type"=3, "Command"="MEAS{Measurement}:GATE:SHOW", "Access"=2, "Range Table"="", "Read Callback"="", "Write Callback"="", "Supported Models"="", "Instrument Options"="", "Flags"=0, "Help"="Indicates the gate area in the source diagram.\n\nAvailable Repeated Capabilities:\nMeasurement: Meas1, Meas2, Meas3, Meas4, Meas5, Meas6, Meas7, Meas8, Meas9, Meas10\r\n\nRemote-control command(s):\nMEASurement<m>:GATE:SHOW"}, {"Level"=3, "Class Only"=FALSE, "Identifier"="RSSCOPE_ATTR_GATING_ZOOM_COUPLING_ENABLED", "Descriptive Name"="Gating Zoom Coupling Enabled", "Data Type"=3, "Command"="MEAS{Measurement}:GATE:ZCO", "Access"=2, "Range Table"="", "Read Callback"="", "Write Callback"="", "Supported Models"="", "Instrument Options"="", "Flags"=0, "Help"="If enabled, the gate area is defined identically to the zoom area for the zoom diagram.\n\nAvailable Repeated Capabilities:\nMeasurement: Meas1, Meas2, Meas3, Meas4, Meas5, Meas6, Meas7, Meas8, Meas9, Meas10\r\n\nRemote-control command(s):\nMEASurement<m>:GATE:ZCOupling"}, {"Level"=3, "Class Only"=FALSE, "Identifier"="RSSCOPE_ATTR_GATING_CURSOR_COUPLING_ENABLED", "Descriptive Name"="Gating Cursor Coupling Enabled", "Data Type"=3, "Command"="MEAS{Measurement}:GATE:CCO", "Access"=2, "Range Table"="", "Read Callback"="", "Write Callback"="", "Supported Models"="", "Instrument Options"="", "Flags"=0, "Help"="Enables the cursor coupling for automatic measurements.\n\nAvailable Repeated Capabilities:\nMeasurement: Meas1, Meas2, Meas3, Meas4, Meas5, Meas6, Meas7, Meas8, Meas9, Meas10\r\n\nRemote-control command(s):\nMEASurement<m>:GATE:CCOupling"}, {"Level"=3, "Class Only"=FALSE, "Identifier"="RSSCOPE_ATTR_GATING_COUPLING_ENABLED", "Descriptive Name"="Gating Coupling Enabled", "Data Type"=3, "Command"="MEAS{Measurement}:GATE:GCO", "Access"=2, "Range Table"="", "Read Callback"="", "Write Callback"="", "Supported Models"="", "Instrument Options"="", "Flags"=0, "Help"="If you enable the gate coupling, the gate settings of the selected measurement are copied to all other measurements. If zoom or cursor coupling is active in a measurement, the zoom size and cursor positions are adjusted.\n\nAvailable Repeated Capabilities:\nMeasurement: Meas1, Meas2, Meas3, Meas4, Meas5, Meas6, Meas7, Meas8, Meas9, Meas10\r\n\nRemote-control command(s):\nMEASurement<m>:GATE:GCOupling"}, {"Level"=3, "Class Only"=FALSE, "Identifier"="RSSCOPE_ATTR_GATING_CURSOR_SET", "Descriptive Name"="Gating Cursor Set", "Data Type"=0, "Command"="MEAS{Measurement}:GATE:CURS", "Access"=2, "Range Table"="RsScope_rngGatingCursorSet", "Read Callback"="", "Write Callback"="", "Supported Models"="", "Instrument Options"="", "Flags"=0, "Help"="Selects the cursor set to be used for measurement gating. The gate area is defined by the cursor lines.\n\nAvailable Repeated Capabilities:\nMeasurement: Meas1, Meas2, Meas3, Meas4, Meas5, Meas6, Meas7, Meas8, Meas9, Meas10\r\n\nRemote-control command(s):\nMEASurement<m>:GATE:CURSor"}, {"Level"=2, "Class Only"=TRUE, "Identifier"="", "Descriptive Name"="Results", "Data Type"=0, "Command"="", "Access"=0, "Range Table"="", "Read Callback"="", "Write Callback"="", "Supported Models"="", "Instrument Options"="", "Flags"=0, "Help"="Queries selected result."}, {"Level"=3, "Class Only"=FALSE, "Identifier"="RSSCOPE_ATTR_READ_MAIN_MEASUREMENT_ACTUAL", "Descriptive Name"="Read Main Measurement Actual", "Data Type"=1, "Command"="MEAS{Measurement}:RES?", "Access"=0, "Range Table"="", "Read Callback"="", "Write Callback"="", 
